vi "_PC_Daemon_Pressurevi.vi"(7 "Function":enum16{"Get reference", "Show graph"}(ring)=enum."Show graph", 8 "error in (no error)":errorcluster) -> (0 "error out":errorcluster, 3 "XY Graph":refnum<vi>)   [LabVIEW 2018]
uses:
  <vilib>/event_ctls.llb/eventvkey.ctl
panel:
  out "Pressure Graph":cluster{timestamp, "Double":dbl}[](graph)
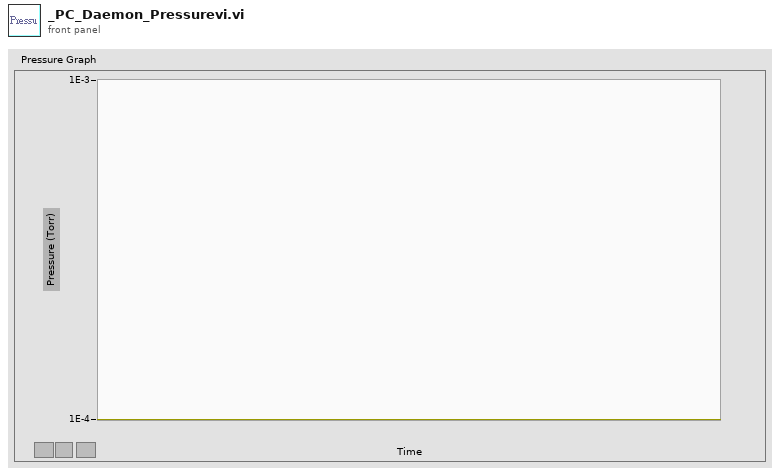
[diagram p1: front panel]
types:
  T1 = typedef "eventvkey.ctl" = enum16{"ASCII", "Enter", "Return", "Shift", "Ctrl", "Alt", "Cmd", "Opt", "Caps", "NumLock", "Clear", "Break", "Up", "Down", "Left", "Right", "Insert", "Delete", "Home", "End", "PageUp", "PageDown", "Escape", "Help", "Pause", "ScrollLock", "F1", "F2", "F3", "F4", "F5", "F6", "F7", "F8", "F9", "F10", "F11", "F12", "F13", "F14", "F15", "F16", "F17", "F18", "F19", "F20", "F21", "F22", "F23", "F24", "Play", "VolumeUp", "VolumeDown", "Mute", "Two Byte Char"}
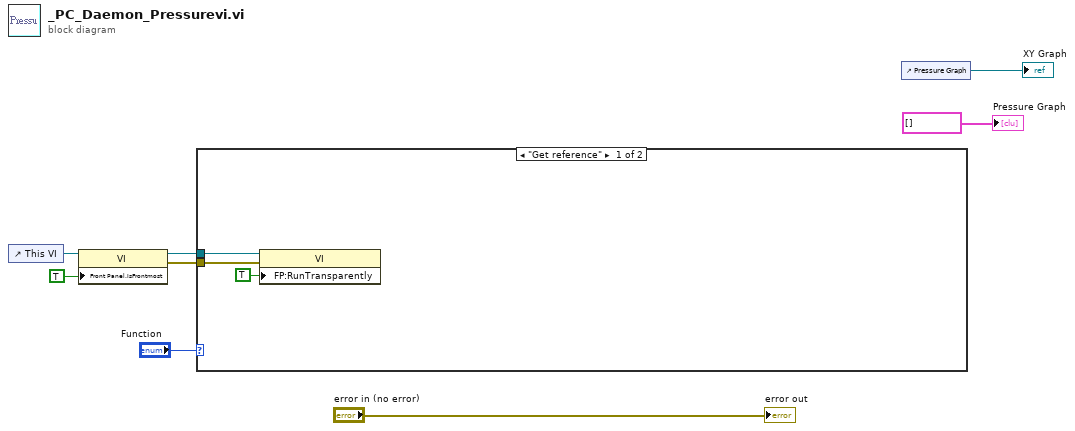
[diagram p0: block diagram]
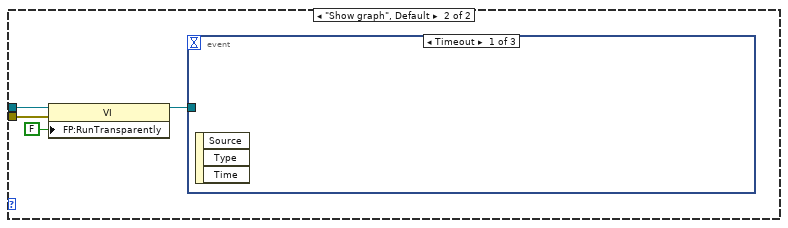
[diagram p2: hidden frame]
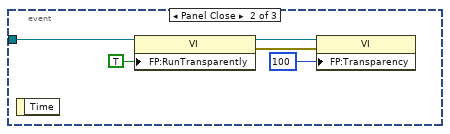
[diagram p3: hidden frame]
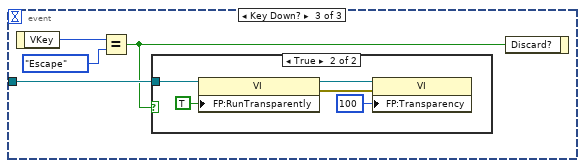
[diagram p4: hidden frame]
diagram:
  n1 = control-ref of="This VI"() -> (w5:refnum<vi>)
  n2 = property class="VI"(reference=w5, "Front Panel.IsFrontmost"=TRUE) -> (reference out=w2:refnum<vi>, error out=w1:errorcluster)  [unwired: 1 in]
  n3 = case shown="\"Get reference\"" "Function" {
    tunnel: w2 -> [w11 w15]
    tunnel: w1 -> [w10 w14]
    frame "Get reference" {
      n4 = property class="VI"(reference=w11, error in=w10, "FP:RunTransparently"=TRUE ("Front Panel Window:Run VI Transparently")) -> ()  [unwired: 2 out]
    }
    frame "Show graph", Default {
      n5 = property class="VI"(reference=w15, error in=w14, "FP:RunTransparently"=FALSE ("Front Panel Window:Run VI Transparently")) -> (reference out=w12:refnum<vi>)  [unwired: 1 out]
      n6 = event shown="[0] Timeout" {
        selector: _ -> [_ _ _]
        dyn-events: _ -> [_ _ _]
        timeout: _ -> [_ _ _]
        tunnel: w12 -> [_ w16 w24]
        event Timeout {
          n7 = event-data() -> ()  [unwired: 1 in, 3 out]
        }
        event Panel Close {
          n8 = event-data() -> ()  [unwired: 1 in, 1 out]
          n9 = property class="VI"(reference=w16, "FP:RunTransparently"=TRUE ("Front Panel Window:Run VI Transparently")) -> (reference out=w20:refnum<vi>, error out=w19:errorcluster)  [unwired: 1 in]
          n10 = property class="VI"(reference=w20, error in=w19, "FP:Transparency"=u8 100 ("Front Panel Window:Transparency")) -> ()  [unwired: 2 out]
        }
        event Key Down? {
          n11 = event-data() -> ("VKey"=w23:T1)  [unwired: 1 in]
          n12 = Equal?(x=w23, y=eventvkey."Escape") -> (x = y?=w21:bool)
          n13 = case shown="True" w21 {
            tunnel: w24 -> [_ w25]
            frame False {
            }
            frame True {
              n14 = property class="VI"(reference=w25, "FP:RunTransparently"=TRUE ("Front Panel Window:Run VI Transparently")) -> (reference out=w29:refnum<vi>, error out=w28:errorcluster)  [unwired: 1 in]
              n15 = property class="VI"(reference=w29, error in=w28, "FP:Transparency"=u8 100 ("Front Panel Window:Transparency")) -> ()  [unwired: 2 out]
            }
          }
          n16 = event-data("Discard?"=w21) -> ()  [unwired: 1 in, 1 out]
        }
      }
    }
  }
  n17 = control-ref of="Pressure Graph"() -> (→"XY Graph":refnum<vi>)
  "Pressure Graph" <- cluster{timestamp, "Double":dbl}[] []
  "error out" <- "error in (no error)"
